vi "Read_Cycling_File.vi"(6 "Total Cycles":i32, 8 "error in (no error)":errorcluster, 11 "Cycling file path In (dialog if empty)":path=path "C:/Sandbox/Git_Sandbox/Tools/MEMS Resistance Char/MEMS_Res_Cycling.txt") -> (0 "error out":errorcluster, 3 "Cycling Cluster":T1)   [LabVIEW 2017]
uses:
  Controls/Cycling_Cluster.ctl
  <vilib>/Utility/file.llb/Read Delimited Spreadsheet (I64).vi
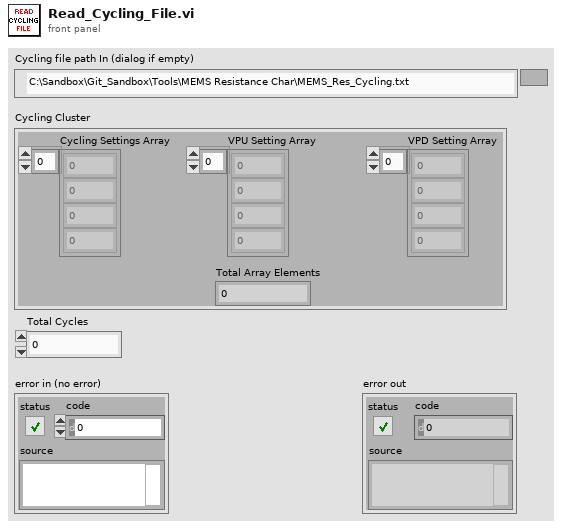
[diagram p1: front panel]
types:
  T1 = typedef "Cycling_Cluster.ctl" = cluster{"Cycling Settings Array":i64[], "VPU Setting Array":i64[], "VPD Setting Array":i64[], "Total Array Elements":i32}
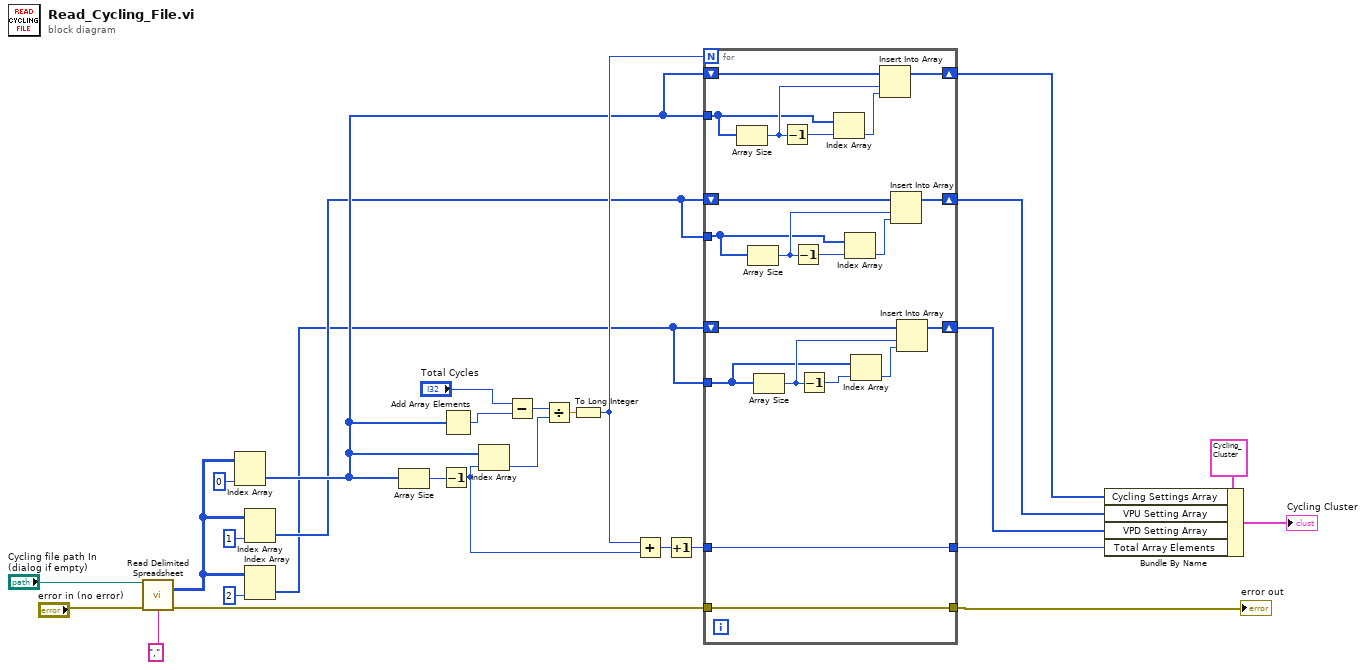
[diagram p0: block diagram]
diagram:
  n1 = call-poly <vilib>:"Read Delimited Spreadsheet.vi"("file path (dialog if empty)"="Cycling file path In (dialog if empty)", "error in (no error)"="error in (no error)", "delimiter (\\t)"="," ("delimiter (\\t)")) -> ("all rows"=w22:i64[][], "error out"=w2:errorcluster)  [unwired: 7 in, 4 out]
  n2 = Index Array(array=w22, index (col)=0 ("disabled index (col)")) -> (element=w10:i64[])  [unwired: 1 in]
  n3 = Index Array(array=w22, index (col)=1 ("disabled index (col)")) -> (element=w9:i64[])  [unwired: 1 in]
  n4 = Index Array(array=w22, index (col)=2 ("disabled index (col)")) -> (element=w8:i64[])  [unwired: 1 in]
  n5 = Array Size(array=w10) -> (size(s)=w15:i32)
  n6 = Decrement(x=w15) -> (x-1=w12:i32)
  n7 = Add Array Elements(numeric array=w10) -> (sum=w18:i64)
  n8 = Index Array(array=w10, index=w12) -> (element=w16:i64)
  n9 = Subtract(x="Total Cycles", y=w18) -> (x-y=w17:i64)
  n10 = Divide(x=w17, y=w16) -> (x/y=w14:dbl)
  n11 = To Long Integer(number=w14) -> (32bit integer=w11:i32)
  n12 = Add(x=w11, y=w12) -> (x+y=w13:i32)
  n13 = Increment(x=w13) -> (x+1=w7:i32)
  n14 = for {
    N: w11 -> [_]
    tunnel: w10 -> [w44]
    shift-right: [w47] -> w5
    shift-left: w10 -> [w46]
    tunnel: w9 -> [w39]
    shift-right: [w37] -> w4
    shift-left: w9 -> [w38]
    shift-right: [w31] -> w3
    shift-left: w8 -> [w33]
    tunnel: w8 -> [w32]
    tunnel: w7 -> [w30]
    tunnel: [w30] -> w6
    tunnel: w2 -> [w29]
    tunnel: [w29] -> w1
    n15 = Array Size(array=w44) -> (size(s)=w48:i32)
    n16 = Array Size(array=w39) -> (size(s)=w40:i32)
    n17 = Array Size(array=w32) -> (size(s)=w36:i32)
    n18 = Decrement(x=w48) -> (x-1=w45:i32)
    n19 = Decrement(x=w40) -> (x-1=w41:i32)
    n20 = Decrement(x=w36) -> (x-1=w35:i32)
    n21 = Index Array(array=w44, index=w45) -> (element=w43:i64)
    n22 = Index Array(array=w39, index=w41) -> (element=w42:i64)
    n23 = Index Array(array=w32, index=w35) -> (element=w34:i64)
    n24 = Insert Into Array(array=w46, index=w48, new element=w43) -> (w47:i64[])
    n25 = Insert Into Array(array=w38, index=w40, new element=w42) -> (w37:i64[])
    n26 = Insert Into Array(array=w33, index=w36, new element=w34) -> (w31:i64[])
  }
  "error out" <- w1
  n27 = Bundle By Name(cluster=T1 {"Cycling Settings Array"=[0, 2, 8, 90, 900, 4000, 5000, 10000, 10000, 10000], "VPU Setting Array"=[0, 0, 0, 0, 0, 0, 0, 0, 0, 0], "VPD Setting Array"=[50, 50, 50, 50, 50, 50, 50, 50, 50, 50], "Total Array Elements"=0} ("Cycling Cluster"), "Cycling Settings Array"=w5, "VPU Setting Array"=w4, "VPD Setting Array"=w3, "Total Array Elements"=w6) -> (→"Cycling Cluster":T1)
